vi "Autonomous Independent.vi"() -> ()   [LabVIEW 2013]
doc: "This VI is called when autonomous begins, and will automatically be terminated when autonomous ends. You can carry out timed or sensor driven robot movement independently without needing to return to the caller."
uses:
  Robot Global Data.vi
panel:
  in  "PID gains":T1={"proportional gain (Kc)"=2.75, "integral time (Ti, min)"=0.0, "derivative time (Td, min)"=0.0} {"derivative time (Td, min)" format="%.3f"; "integral time (Ti, min)" format="%.3f"; "proportional gain (Kc)" format="%.3f"}
  # "Side? it true when hot goal is right\nand false when it is left"
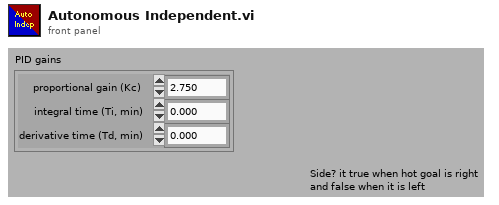
[diagram p1: front panel]
types:
  T1 = cluster{"proportional gain (Kc)":dbl, "integral time (Ti, min)":dbl, "derivative time (Td, min)":dbl}
  T2 = typedef "WPI_CameraDevRef.ctl" = cluster{"Camera Address":string, "CameraStatus":errorcluster, "Acquire Image Notifier":refnum<notifier>}
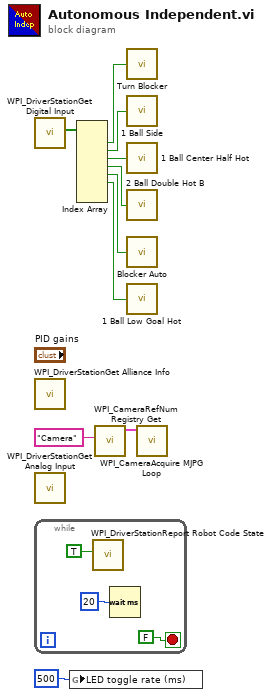
[diagram p0: block diagram]
diagram:
  n1 = call <vilib>:"WPI_DriverStationGet Digital Input.vi"() -> ("Driver Station Digital Input (1-8)"=w10:bool[])  [unwired: 11 out]
  n2 = call <vilib>:"WPI_DriverStationGet Alliance Info.vi"() -> ()  [unwired: 12 out]
  n3 = call <vilib>:"WPI_DriverStationGet Analog Input.vi"() -> ()  [unwired: 12 out]
  n4 = while {
    stop <- FALSE stop-if-true
    n5 = call <vilib>:"WPI_DriverStationReport Robot Code State.vi"("Autonomous"=TRUE) -> ()  [unwired: 10 in, 1 out]
    n6 = Wait (ms)(milliseconds to wait=u32 20) -> ()  [unwired: 1 out]
  }
  n7 = global write "Robot Global Data.vi" "LED toggle rate (ms)"(u32 500 ("LED ms toggle rate")) -> ()
  n8 = Index Array(array=w10) -> (element #1=w2:bool, element #2=w1:bool, element #3=w6:bool, element #4=w4:bool, element #5=w3:bool, element #6=w5:bool)  [unwired: 8 in, 2 out]
  n9 = call <vilib>:"WPI_CameraRefNum Registry Get.vi"("refnum name"="Camera") -> ("CameraDevRef"=w7:T2)  [unwired: 9 in, 1 out]
  n10 = call "Turn Blocker.vi"("Run?"=w2) -> ()  [unwired: 1 in]
  n11 = call "1 Ball Side.vi"("Run?"=w1) -> ()  [unwired: 1 in]
  n12 = call "1 Ball Center Half Hot.vi"("Run?"=w6) -> ()  [unwired: 1 out]
  n13 = call "2 Ball Double Hot B.vi"("Run?"=w4) -> ()  [unwired: 1 out]
  n14 = call "Blocker Auto.vi"("Run?"=w3) -> ()  [unwired: 1 out]
  n15 = call "1 Ball Low Goal Hot.vi"("Run?"=w5) -> ()  [unwired: 1 out]
  n16 = call <vilib>:"WPI_CameraAcquire MJPG Loop.vi"("CameraDevRef"=w7) -> ()  [unwired: 11 in]
